vi "Value Strings.vi"(8 "error in (no error)":errorcluster, 11 "Group BOOL in":refnum<class "Group BOOL.lvclass">) -> (0 "error out":errorcluster, 1 "Timestamp":dbl[](array[numeric]), 2 "Value Strings":string[](array[string]), 3 "Group BOOL out":refnum<class "Group BOOL.lvclass">)   [LabVIEW 2020, in "Vecto.lvlib" / "Group BOOL.lvclass"]
uses:
  Group BOOL.lvclass
  Group BOOL.lvclass/Group BOOL.ctl
  Vecto.lvlib
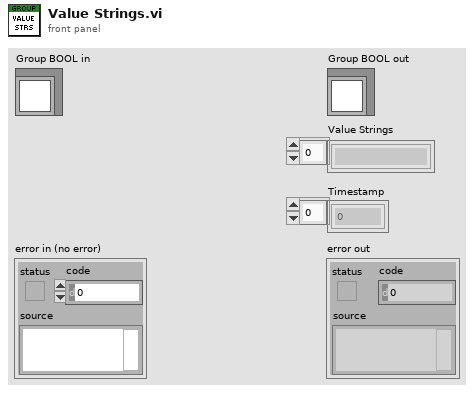
[diagram p1: front panel]
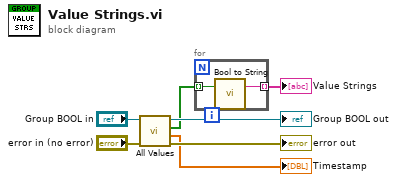
[diagram p0: block diagram]
diagram:
  n1 = call "All Values.vi"("error in (no error)"="error in (no error)", "Group BOOL in"="Group BOOL in") -> ("error out"=→"error out":errorcluster, "Timestamp"=→"Timestamp":dbl[], "Scaled"=w2:bool[], "Group BOOL out"=→"Group BOOL out":refnum<class "Group BOOL.lvclass">)  [unwired: 5 in, 1 out]
  n2 = for {
    tunnel: w2 -> [w9] mode=indexing
    tunnel: [w8] -> w1 mode=indexing
    n3 = call "Bool to String.vi"("Bool"=w9) -> ("String"=w8:string)  [unwired: 2 in]
  }
  "Value Strings" <- w1
